vi "Asynchronous Logging Loop.vi"(10 "Input Data":T7 {"File Logging Specs"."File Node Ref" format="%.0x"}) -> ()   [LabVIEW 2019, in "Embedded Data Logger Engine.lvlib"]
uses:
  Embedded Data Logger Engine.lvlib
  File Logging Specification.ctl
  Group Logging Specification.ctl
  Group Buffer Data.ctl
  Property Specification.ctl
  <vilib>/NI VeriStand/Custom Device API/Custom Device Item Ref.ctl
  Shared/Segment Files By.ctl
  Asynchronous Logging Loop State.ctl
  Add to Flushed Data Size.vi
  <vilib>/NI VeriStand/Custom Device API/Custom Device API.lvlib
  Shared/Embedded Data Logger Shared.lvlib
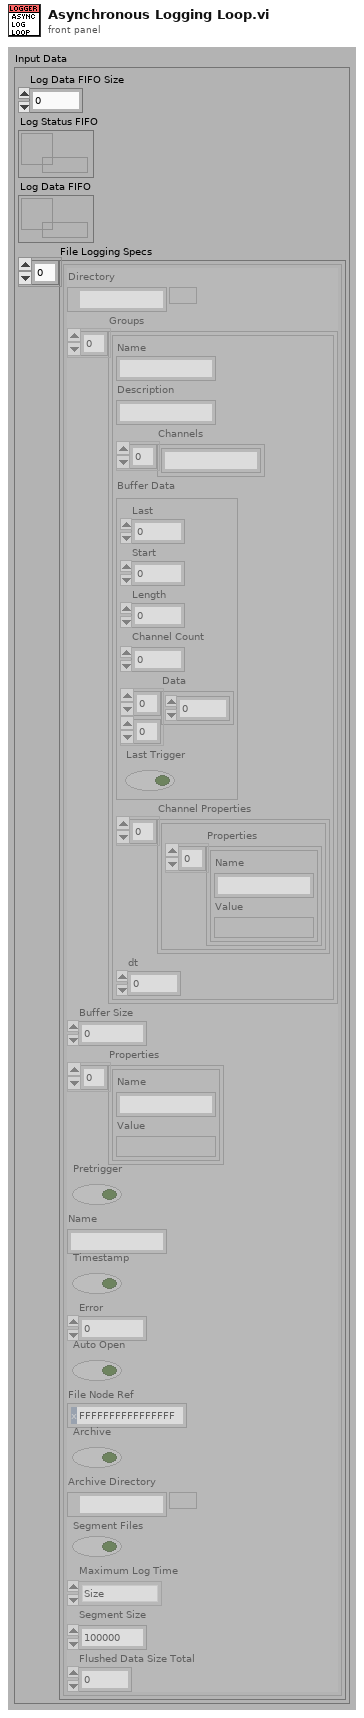
[diagram p1: front panel]
types:
  T1 = typedef "Embedded Data Logger Engine.lvlib/File Logging Specification.ctl" = cluster{"Directory":path, "Groups":T2[], "Buffer Size":i32, "Properties":T4[], "Pretrigger":bool, "Name":string, "Timestamp":bool, "Error":i32, "Auto Open":bool, "File Node Ref":T5, "Archive":bool, "Archive Directory":path, "Segment Files":bool, "Segment Files By":T6, "Segment Size":u32, "Flushed Data Size Total":u32}
  T2 = typedef "Embedded Data Logger Engine.lvlib/Group Logging Specification.ctl" = cluster{"Name":string, "Description":string, "Channels":string[], "Buffer Data":T3, "Channel Properties":cluster{"Properties":T4[]}[], "dt":dbl}
  T3 = typedef "Embedded Data Logger Engine.lvlib/Group Buffer Data.ctl" = cluster{"Last":i32, "Start":i32, "Length":i32, "Channel Count":i32, "Data":dbl[][], "Last Trigger":bool}
  T4 = typedef "Embedded Data Logger Engine.lvlib/Property Specification.ctl" = cluster{"Name":string, "Value":variant}
  T5 = typedef "Custom Device API.lvlib/Custom Device Item Ref.ctl" = u64
  T6 = typedef "Embedded Data Logger Shared.lvlib/Segment Files By.ctl" = enum16{"Time", "Size"}
  T7 = cluster{"Log Data FIFO Size":i32, "Log Status FIFO":refnum<k33>, "Log Data FIFO":refnum<k33>, "File Logging Specs":T1[]}
  T8 = typedef "Embedded Data Logger Engine.lvlib/Asynchronous Logging Loop State.ctl" = enum16{"Initialize", "Check Cmd", "Log Data", "Open File", "Close File", "Shut Down", "Open File then Log Data"}
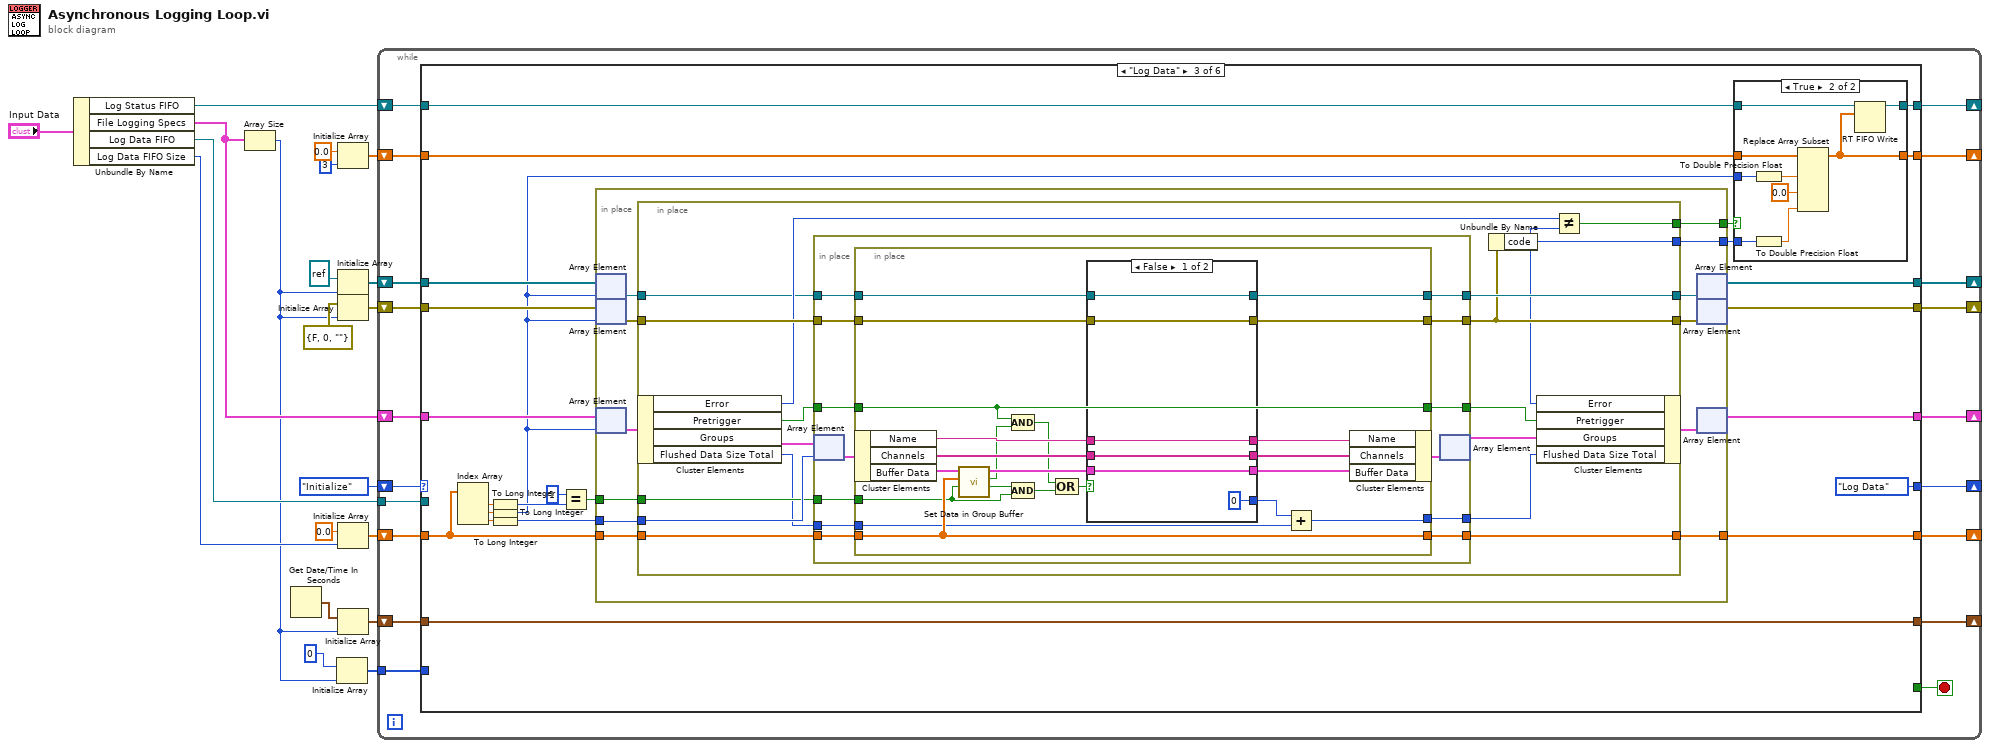
[diagram p0: block diagram]
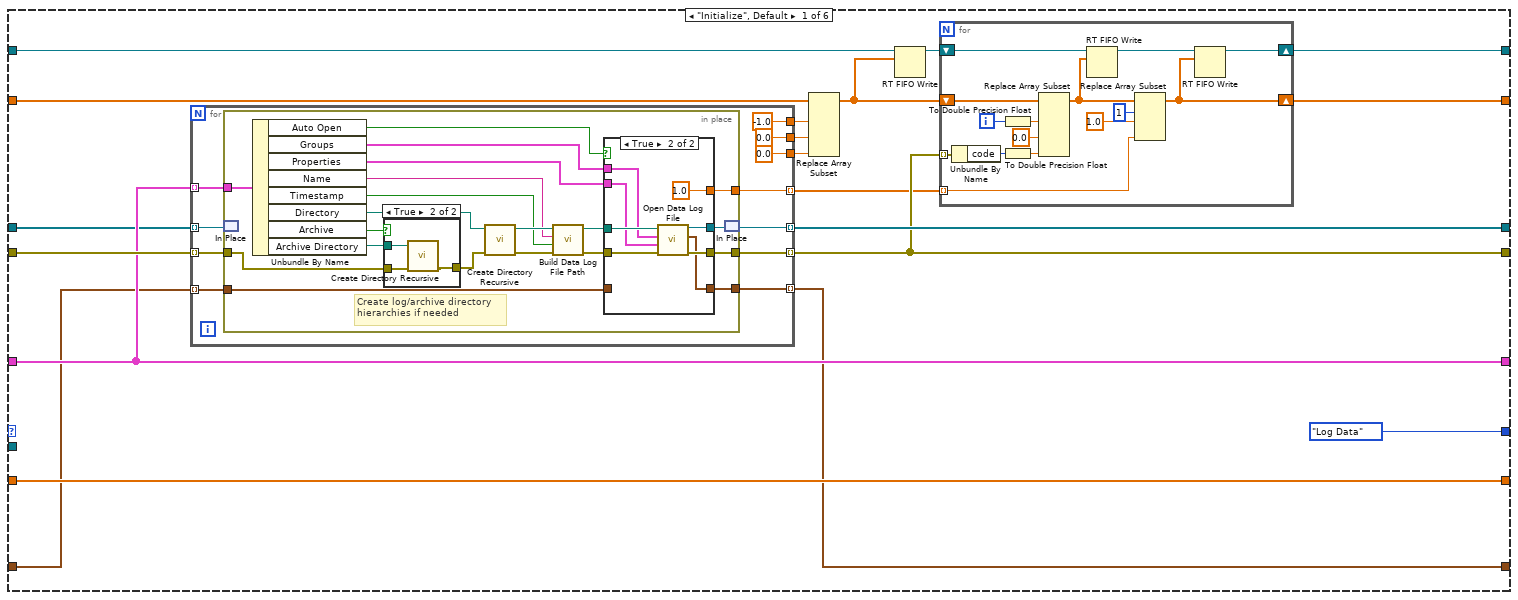
[diagram p2: hidden frame]
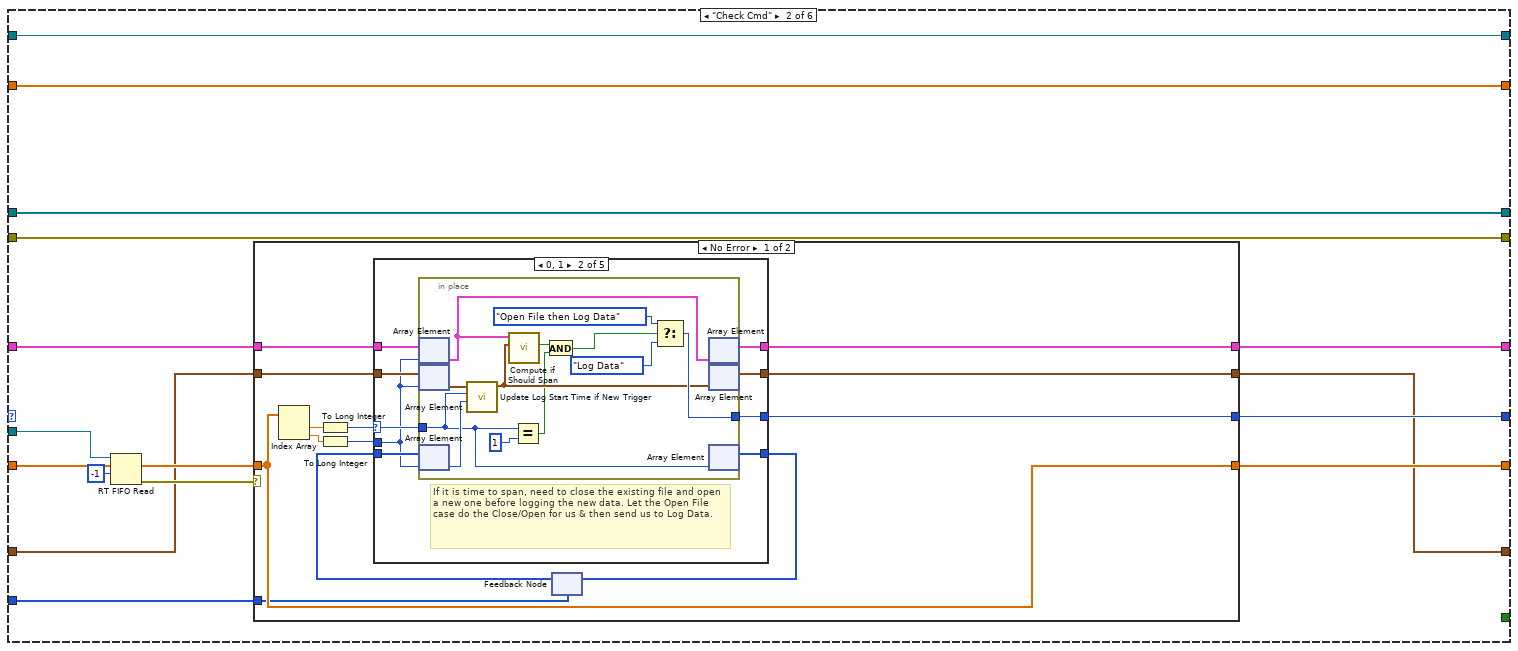
[diagram p5: hidden frame]
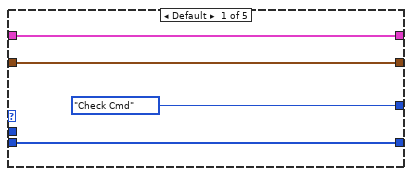
[diagram p6: hidden frame]
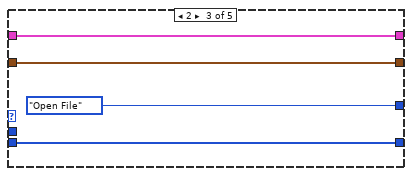
[diagram p7: hidden frame]
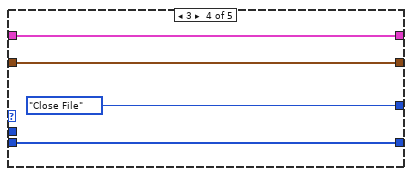
[diagram p8: hidden frame]
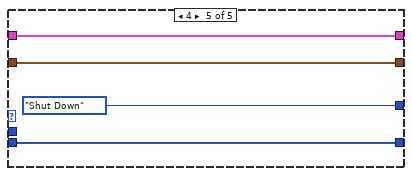
[diagram p9: hidden frame]
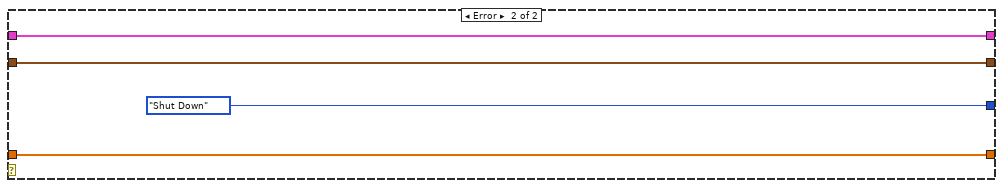
[diagram p10: hidden frame]
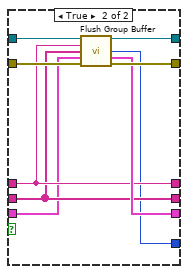
[diagram p11: hidden frame]
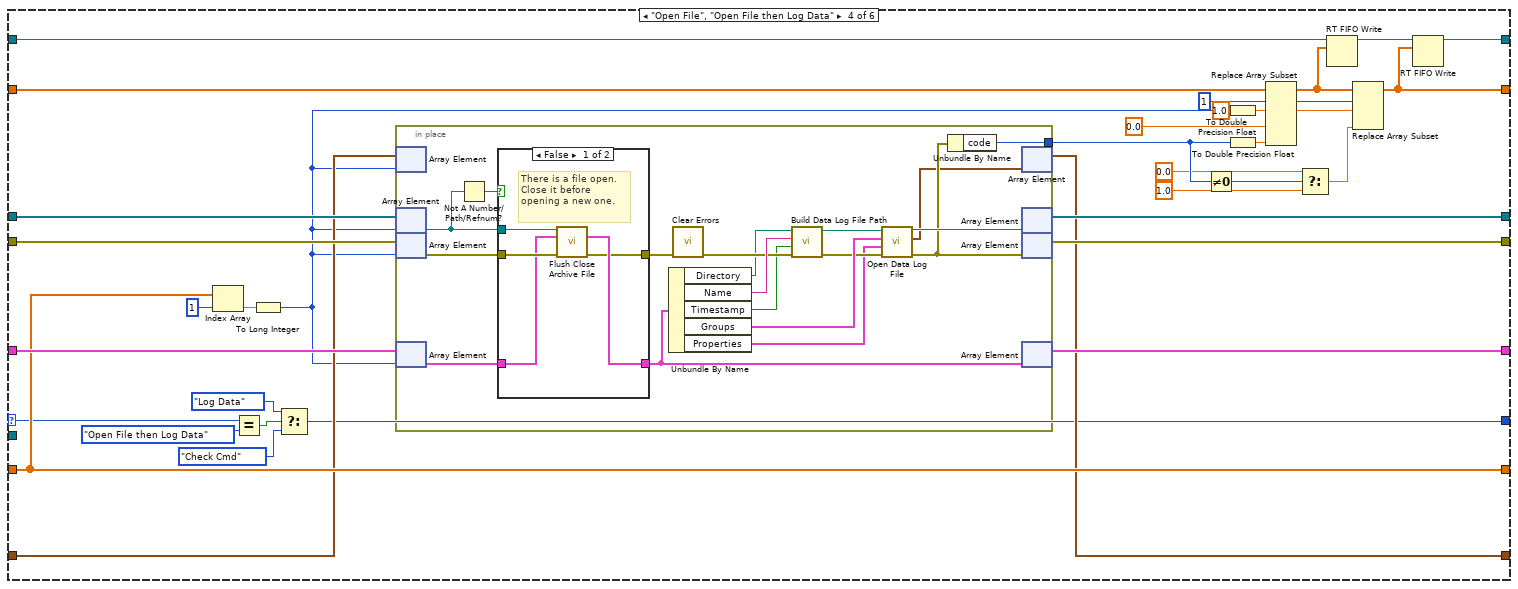
[diagram p13: hidden frame]
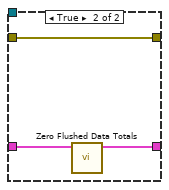
[diagram p14: hidden frame]
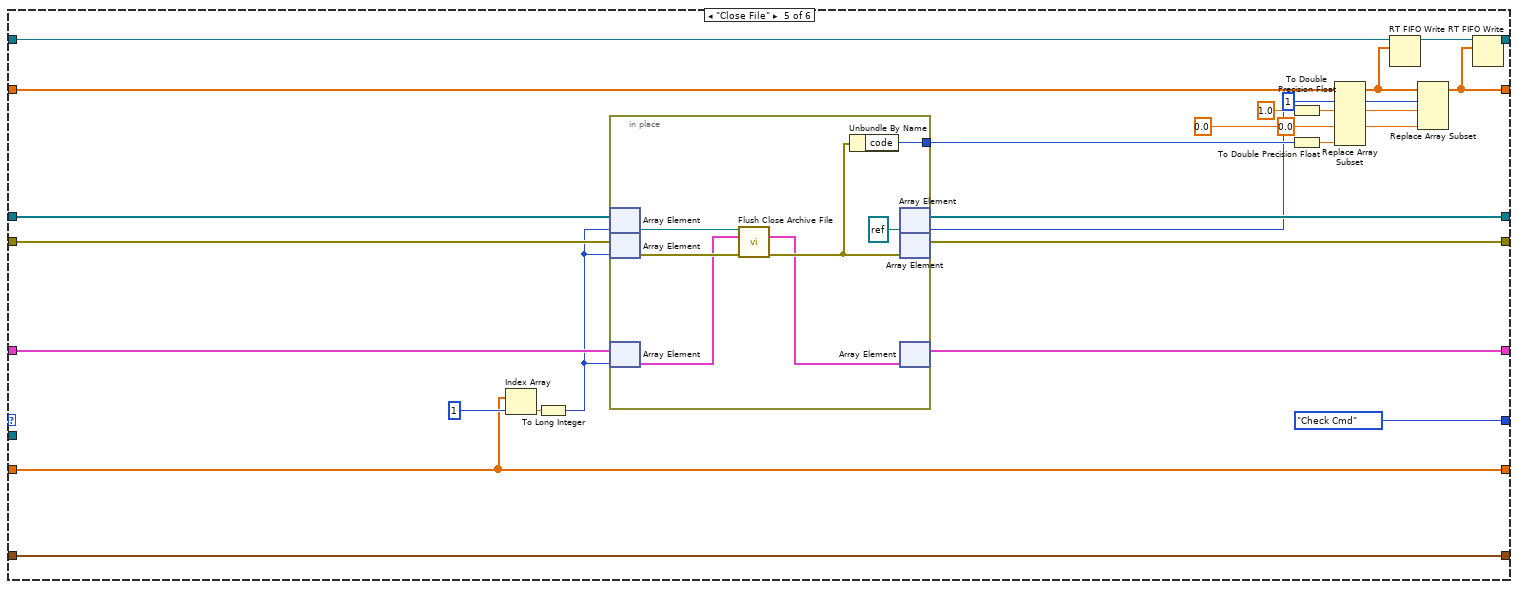
[diagram p15: hidden frame]
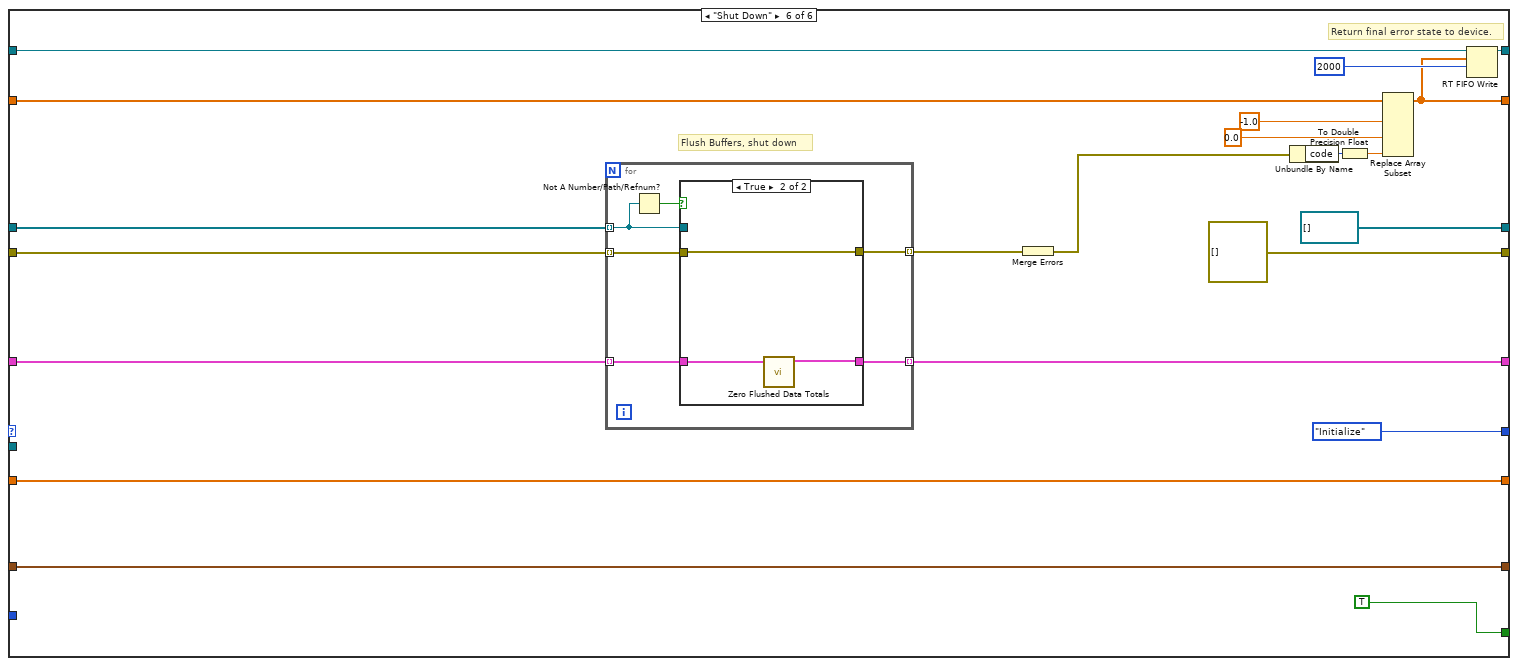
[diagram p16: hidden frame]
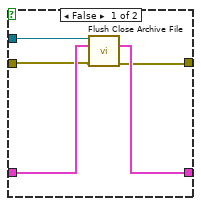
[diagram p17: hidden frame]
diagram:
  n1 = Unbundle By Name("Input Data") -> ("Log Status FIFO"=w14:refnum<k33>, "File Logging Specs"=w11:T1[], "Log Data FIFO"=w16:refnum<k33>, "Log Data FIFO Size"=w17:i32)
  n2 = Array Size(array=w11) -> (size(s)=w4:i32)
  n3 = Get Date/Time In Seconds() -> (seconds since 1Jan1904=w1:timestamp)
  n4 = Initialize Array(0 ("y"), w4) -> (w2:i32[])
  n5 = Initialize Array(0.0 ("element"), 3 ("dimension size")) -> (w6:dbl[])
  n6 = Initialize Array(refnum<k34> refnum ("TDMS File Ref out"), w4) -> (w9:refnum<k34>[])
  n7 = Initialize Array(errorcluster {"status"=FALSE, "code"=0, "source"=""} ("error in (no error)"), w4) -> (w12:errorcluster[])
  n8 = Initialize Array(0.0 ("element"), w17) -> (w19:dbl[])
  n9 = Initialize Array(w1, w4) -> (w5:timestamp[])
  n10 = while {
    tunnel: w16 -> [w39]
    shift-right: [w35] -> _
    shift-left: w19 -> [w38]
    shift-right: [w29] -> _
    shift-left: w9 -> [w28]
    shift-right: [w32] -> _
    shift-left: w11 -> [w33]
    shift-right: [w27] -> _
    shift-left: w14 -> [w26]
    shift-right: [w31] -> _
    shift-left: w12 -> [w30]
    shift-right: [w34] -> _
    shift-left: Asynchronous_Logging_Loop_State."Initialize" ("State") -> [w37]
    shift-right: [w24] -> _
    shift-left: w6 -> [w25]
    shift-right: [w22] -> _
    shift-left: w5 -> [w23]
    tunnel: w2 -> [w21]
    stop <- w36 stop-if-true
    n11 = case shown="\"Log Data\"" w37 {
      selector: w37 -> [_ _ _ w309 _ _]
      tunnel: w39 -> [_ w134 _ _ _ _]
      tunnel: w38 -> [w57 w120 w207 w328 w381 w413]
      tunnel: [_ _ _ _ _ TRUE] -> w36
      tunnel: [w57 w126 w196 w328 w381 w413] -> w35
      tunnel: [Asynchronous_Logging_Loop_State."Log Data" ("State") w125 Asynchronous_Logging_Loop_State."Log Data" ("State") w305 Asynchronous_Logging_Loop_State."Check Cmd" ("State") Asynchronous_Logging_Loop_State."Initialize" ("State")] -> w34
      tunnel: w33 -> [w54 w121 w202 w330 w367 w398]
      tunnel: [w54 w122 w197 w329 w364 w397] -> w32
      tunnel: [w51 w130 w198 w331 w383 errorcluster[] []] -> w31
      tunnel: w30 -> [w58 w130 w208 w332 w384 w414]
      tunnel: [w55 w129 w200 w333 w385 refnum<k34>[] []] -> w29
      tunnel: w28 -> [w50 w129 w209 w334 w386 w415]
      tunnel: [w45 w128 w199 w322 w372 w406] -> w27
      tunnel: w26 -> [w53 w128 w212 w324 w379 w399]
      tunnel: w25 -> [w49 w127 w191 w327 w378 w402]
      tunnel: [w44 w127 w192 w320 w368 w403] -> w24
      tunnel: w23 -> [w41 w123 w189 w311 w363 w396]
      tunnel: [w40 w124 w189 w310 w363 w396] -> w22
      tunnel: w21 -> [_ w119 _ _ _ _]
      frame "Initialize", Default {
        n12 = for {
          tunnel: w54 -> [w84] mode=indexing
          tunnel: [w81] -> w55 mode=indexing
          tunnel: [w82] -> w51 mode=indexing
          tunnel: w58 -> [w83] mode=indexing
          tunnel: w50 -> [w80] mode=indexing
          tunnel: [-1.0 ("new element/subarray")] -> w48
          tunnel: [0.0 ("new element/subarray")] -> w47
          tunnel: [w77] -> w43 mode=indexing
          tunnel: [0.0 ("new element/subarray")] -> w42
          tunnel: w41 -> [w74] mode=indexing
          tunnel: [w75] -> w40 mode=indexing
          n13 = in-place {
            in-place-border: w84 -> [w104]
            in-place-border: w83 -> [w90]
            in-place-border: [w96] -> w82
            in-place-border: [w93] -> w77
            in-place-border: [w86] -> w75
            in-place-border: w74 -> [w85]
            # "Create log/archive directory hierarchies if needed"
            n14 = in-place-match #1(w80) -> ()  [unwired: 1 out]
            n15 = Unbundle By Name(w104) -> ("Auto Open"=w94:bool, "Groups"=w97:T2[], "Properties"=w98:T4[], "Name"=w101:string, "Timestamp"=w100:bool, "Directory"=w88:path, "Archive"=w92:bool, "Archive Directory"=w89:path)
            n16 = case shown="True" w92 {
              tunnel: [w105 w108] -> w91
              tunnel: w90 -> [w105 w107]
              tunnel: w89 -> [_ w106]
              frame False {
              }
              frame True {
                n17 = call <vilib>:"Create Directory Recursive.vi"("error in (no error)"=w107, "directory"=w106) -> ("error out"=w108:errorcluster)  [unwired: 1 in, 4 out]
              }
            }
            n18 = call <vilib>:"Create Directory Recursive.vi"("error in (no error)"=w91, "directory"=w88) -> ("error out"=w103:errorcluster, "directory copy"=w102:path)  [unwired: 1 in, 3 out]
            n19 = call "Build Data Log File Path.vi"("error in (no error)"=w103, "Timestamp"=w100, "Name"=w101, "Log File Directory"=w102) -> ("error out"=w99:errorcluster, "appended path"=w87:path)  [unwired: 6 in]
            n20 = case shown="True" w94 {
              tunnel: w99 -> [w110 w118]
              tunnel: w87 -> [_ w117]
              tunnel: w98 -> [_ w116]
              tunnel: w97 -> [_ w115]
              tunnel: [w110 w114] -> w96
              tunnel: [_ w113] -> w95
              tunnel: [_ 1.0 ("new element/subarray")] -> w93
              tunnel: [w109 w111] -> w86
              tunnel: w85 -> [w109 _]
              frame False {
              }
              frame True {
                n21 = call "Open Data Log File.vi"("error in"=w118, "File Properties"=w116, "Channel Groups"=w115, "Data Log File Path"=w117) -> ("error out"=w114:errorcluster, "File Start Time"=w111:timestamp, "tdms file out"=w113:refnum<k34>)  [unwired: 5 in]
              }
            }
            n22 = in-place-match #1(w95) -> (w81:refnum<k34>)
          }
        }
        n23 = Replace Array Subset(array=w49, new element #1=w48, new element #2=w47, new element #3=w42) -> (w46:dbl[])  [unwired: 3 in]
        n24 = RT FIFO Write(0:w53, 1:w46) -> (8:w52:refnum<k33>)  [unwired: 2 in, 4 out]
        n25 = for {
          shift-right: [w63] -> w45
          shift-left: w52 -> [w73]
          tunnel: w51 -> [w71] mode=indexing
          shift-right: [w59] -> w44
          shift-left: w46 -> [w69]
          tunnel: w43 -> [w60] mode=indexing
          i -> [w72]
          n26 = Unbundle By Name(w71) -> ("code"=w70:i32)
          n27 = To Double Precision Float(number=w72) -> (double precision float=w66:dbl)
          n28 = To Double Precision Float(number=w70) -> (double precision float=w68:dbl)
          n29 = Replace Array Subset(array=w69, new element #1=w66, new element #2=0.0 ("new element/subarray"), new element #3=w68) -> (w67:dbl[])  [unwired: 3 in]
          n30 = RT FIFO Write(0:w73, 1:w67) -> (8:w64:refnum<k33>)  [unwired: 2 in, 4 out]
          n31 = Replace Array Subset(array=w67, new element #1=1.0 ("new element/subarray"), index #1=1 ("index"), new element #2=w60) -> (w59:dbl[])  [unwired: 1 in]
          n32 = RT FIFO Write(0:w64, 1:w59) -> (8:w63:refnum<k33>)  [unwired: 2 in, 4 out]
        }
      }
      frame "Check Cmd" {
        n33 = RT FIFO Read(0:w134, 1:w120, 2:-1 ("timeout in ms (0)")) -> (9:w131:dbl[], 11:w132:errorcluster)  [unwired: 1 in, 3 out]
        n34 = case shown="No Error" w132 {
          tunnel: [w138 w187] -> w126
          tunnel: w131 -> [w138 w187]
          tunnel: [w145 Asynchronous_Logging_Loop_State."Shut Down" ("State")] -> w125
          tunnel: w121 -> [w142 w186]
          tunnel: w123 -> [w141 w185]
          tunnel: [w140 w185] -> w124
          tunnel: [w139 w186] -> w122
          tunnel: w119 -> [w137 _]
          frame No Error {
            n35 = Index Array(array=w138) -> (element #1=w147:dbl, element #2=w144:dbl)  [unwired: 2 in]
            n36 = To Long Integer(number=w147) -> (32bit integer=w146:i32)
            n37 = To Long Integer(number=w144) -> (32bit integer=w143:i32)
            n38 = feedback #2(w137) -> (w136:i32[])
            n39 = case shown="0, 1" w146 {
              selector: w146 -> [_ w155 _ _ _]
              tunnel: [Asynchronous_Logging_Loop_State."Check Cmd" ("State") w158 Asynchronous_Logging_Loop_State."Open File" ("State") Asynchronous_Logging_Loop_State."Close File" ("State") Asynchronous_Logging_Loop_State."Shut Down" ("State")] -> w145
              tunnel: w143 -> [_ w153 _ _ _]
              tunnel: w142 -> [w149 w160 w175 w178 w182]
              tunnel: w141 -> [w150 w159 w174 w179 w183]
              tunnel: [w150 w157 w174 w179 w183] -> w140
              tunnel: [w149 w156 w175 w178 w182] -> w139
              tunnel: w136 -> [w148 w154 w173 w177 w181]
              tunnel: [w148 w152 w173 w177 w181] -> w135
              frame Default {
              }
              frame 0, 1 {
                # "If it is time to span, need to close the existing file and open a new one before logging the new data. Let the Open File case do the Close/Open for us & then send us to Log Data."
                n40 = in-place {
                  in-place-border: [w170] -> w158
                  in-place-border: w155 -> [w161]
                  n41 = in-place-array #3(w160, w153) -> (w169:T1)
                  n42 = in-place-array #4(w159, w153) -> (w166:timestamp)
                  n43 = in-place-array #5(w154, w153) -> (w162:i32)
                  n44 = call "Update Log Start Time if New Trigger.vi"("Previous Trigger Value"=w162, "Current Trigger Value"=w161, "Previous Log Trigger Time"=w166) -> ("Current Log Trigger Time"=w165:timestamp)  [unwired: 8 in]
                  n45 = call "Compute if Should Span.vi"("Log Start Time"=w165, "File Log Specification"=w169) -> ("Span File"=w168:bool)  [unwired: 9 in]
                  n46 = Equal?(x=w161, y=1) -> (x = y?=w163:bool)
                  n47 = And(x=w168, y=w163) -> (x .and. y?=w167:bool)
                  n48 = Select(t=Asynchronous_Logging_Loop_State."Open File then Log Data" ("State"), s=w167, f=Asynchronous_Logging_Loop_State."Log Data" ("State")) -> (s? t:f=w170:T8)
                  n49 = in-place-array #3(w169) -> (w156:T1[])  [unwired: 1 out]
                  n50 = in-place-array #4(w165) -> (w157:timestamp[])  [unwired: 1 out]
                  n51 = in-place-array #5(w161) -> (w152:i32[])  [unwired: 1 out]
                }
              }
              frame 2 {
              }
              frame 3 {
              }
              frame 4 {
              }
            }
            n52 = feedback-in #2(w135) -> ()
          }
          frame Error {
          }
        }
      }
      frame "Log Data" {
        n53 = Index Array(array=w207) -> (element #1=w206:dbl, element #2=w205:dbl, element #3=w204:dbl)  [unwired: 3 in]
        n54 = To Long Integer(number=w206) -> (32bit integer=w203:i32)
        n55 = To Long Integer(number=w205) -> (32bit integer=w190:i32)
        n56 = To Long Integer(number=w204) -> (32bit integer=w201:i32)
        n57 = Equal?(x=1, y=w203) -> (x = y?=w210:bool)
        n58 = in-place {
          in-place-border: w207 -> [w224]
          in-place-border: w201 -> [w223]
          in-place-border: w210 -> [w221]
          in-place-border: [w218] -> w196
          in-place-border: [w215] -> w194
          in-place-border: [w214] -> w193
          n59 = in-place-array #6(w209, w190) -> (w220:refnum<k34>)
          n60 = in-place-array #7(w208, w190) -> (w217:errorcluster)
          n61 = in-place-array #8(w202, w190) -> (w222:T1)
          n62 = in-place {
            in-place-border: w224 -> [w239]
            in-place-border: w223 -> [w238]
            in-place-border: w221 -> [w235]
            in-place-border: w217 -> [w241]
            in-place-border: [w229] -> w216
            in-place-border: w220 -> [w234]
            in-place-border: [w233] -> w219
            in-place-border: [w232] -> w218
            in-place-border: [w228] -> w215
            in-place-border: [w227] -> w214
            n63 = in-place-cluster #9(w222) -> ("Error"=w240:i32, "Pretrigger"=w231:bool, "Groups"=w237:T2[], "Flushed Data Size Total"=w226:u32)
            n64 = in-place {
              in-place-border: w239 -> [w254]
              in-place-border: w235 -> [w251]
              in-place-border: w241 -> [w250]
              in-place-border: [w249] -> w229
              in-place-border: w234 -> [w248]
              in-place-border: [w247] -> w233
              in-place-border: [w246] -> w232
              in-place-border: w231 -> [w245]
              in-place-border: [w244] -> w230
              in-place-border: w226 -> [w243]
              in-place-border: [w242] -> w225
              n65 = in-place-array #10(w237, w238) -> (w253:T2)
              n66 = in-place {
                in-place-border: w254 -> [w264]
                in-place-border: w251 -> [w263]
                in-place-border: w250 -> [w276]
                in-place-border: [w270] -> w249
                in-place-border: w248 -> [w265]
                in-place-border: [w266] -> w247
                in-place-border: [w264] -> w246
                in-place-border: w245 -> [w259]
                in-place-border: [w259] -> w244
                in-place-border: w243 -> [w257]
                in-place-border: [w256] -> w242
                n67 = in-place-cluster #11(w253) -> ("Name"=w271:string, "Channels"=w269:string[], "Buffer Data"=w275:T3)
                n68 = call "Set Data in Group Buffer.vi"("New Trigger"=w263, "Data in"=w264, "Group Buffer Data in"=w275) -> ("Buffer Full"=w274:bool, "Flush Pretrigger Data"=w262:bool, "Group Buffer Data out"=w272:T3)  [unwired: 6 out]
                n69 = Compound Arithmetic op=AND(w259, w262) -> (w260:bool)
                n70 = Compound Arithmetic op=AND(w274, w263) -> (w273:bool)
                n71 = Compound Arithmetic op=OR(w260, w273) -> (w261:bool)
                n72 = case shown="False" w261 {
                  tunnel: w272 -> [w282 w284]
                  tunnel: w271 -> [w280 w286]
                  tunnel: [w282 w289] -> w258
                  tunnel: w276 -> [w281 w291]
                  tunnel: [w281 w290] -> w270
                  tunnel: w269 -> [w279 w285]
                  tunnel: [w280 w286] -> w268
                  tunnel: [w279 w285] -> w267
                  tunnel: [w278 w287] -> w266
                  tunnel: w265 -> [w278 w288]
                  tunnel: [u32 0 ("Flushed Data Size") w283] -> w255
                  frame False {
                  }
                  frame True {
                    n73 = call "Flush Group Buffer.vi"("TDMS File Ref in"=w288, "Group Name"=w286, "Channels"=w285, "Group Buffer Data in"=w284, "error in (no error)"=w291) -> ("TDMS File Ref out"=w287:refnum<k34>, "Flushed Data Size"=w283:u32, "Group Buffer Data out"=w289:T3, "error out"=w290:errorcluster)  [unwired: 1 in, 6 out]
                  }
                }
                n74 = Add(x=w255, y=w257) -> (x+y=w256:u32)
                n75 = in-place-cluster #11("Name"=w268, "Channels"=w267, "Buffer Data"=w258) -> (w252:T2)
              }
              n76 = in-place-array #10(w252) -> (w236:T2[])  [unwired: 1 out]
            }
            n77 = Unbundle By Name(w229) -> ("code"=w228:i32)
            n78 = in-place-cluster #9("Error"=w228, "Pretrigger"=w230, "Groups"=w236, "Flushed Data Size Total"=w225) -> (w213:T1)
            n79 = Not Equal?(x=w240, y=w228) -> (x != y?=w227:bool)
          }
          n80 = in-place-array #6(w219) -> (w200:refnum<k34>[])  [unwired: 1 out]
          n81 = in-place-array #7(w216) -> (w198:errorcluster[])  [unwired: 1 out]
          n82 = in-place-array #8(w213) -> (w197:T1[])  [unwired: 1 out]
        }
        n83 = case shown="True" w193 {
          tunnel: w212 -> [w293 w302]
          tunnel: w190 -> [_ w301]
          tunnel: [w293 w300] -> w199
          tunnel: w194 -> [_ w299]
          tunnel: [w292 w297] -> w192
          tunnel: w191 -> [w292 w298]
          frame False {
          }
          frame True {
            n84 = To Double Precision Float(number=w301) -> (double precision float=w295:dbl)
            n85 = To Double Precision Float(number=w299) -> (double precision float=w296:dbl)
            n86 = Replace Array Subset(array=w298, new element #1=w295, new element #2=0.0 ("new element/subarray"), new element #3=w296) -> (w297:dbl[])  [unwired: 3 in]
            n87 = RT FIFO Write(0:w302, 1:w297) -> (8:w300:refnum<k33>)  [unwired: 2 in, 4 out]
          }
        }
      }
      frame "Open File", "Open File then Log Data" {
        n88 = Index Array(array=w328, index=1) -> (element=w336:dbl)
        n89 = Equal?(x=w309, y=Asynchronous_Logging_Loop_State."Open File then Log Data" ("State")) -> (x = y?=w304:bool)
        n90 = To Long Integer(number=w336) -> (32bit integer=w303:i32)
        n91 = Select(t=Asynchronous_Logging_Loop_State."Log Data" ("State"), s=w304, f=Asynchronous_Logging_Loop_State."Check Cmd" ("State")) -> (s? t:f=w305:T8)
        n92 = in-place {
          in-place-border: [w348] -> w316
          n93 = in-place-array #12(w311, w303) -> ()  [unwired: 1 out]
          n94 = in-place-array #13(w334, w303) -> (w343:refnum<k34>)
          n95 = in-place-array #14(w332, w303) -> (w350:errorcluster)
          n96 = in-place-array #15(w330, w303) -> (w341:T1)
          n97 = Not A Number/Path/Refnum?(number/path/refnum=w343) -> (NaN/Path/Refnum?=w342:bool)
          n98 = case shown="False" w342 {
            tunnel: w350 -> [w358 w362]
            tunnel: [w355 w362] -> w349
            tunnel: w343 -> [w359 _]
            tunnel: [w356 w360] -> w337
            tunnel: w341 -> [w357 w361]
            frame False {
              # "There is a file open. Close it before opening a new one."
              n99 = call "Flush Close Archive File.vi"("TDMS File Refnum In"=w359, "File Log Spec In"=w357, "error in"=w358) -> ("File Log Spec Out"=w356:T1, "error out"=w355:errorcluster)  [unwired: 11 in]
            }
            frame True {
              n100 = call "Zero Flushed Data Totals.vi"("File Log Spec in"=w361) -> ("File Log Spec out"=w360:T1)  [unwired: 10 in]
            }
          }
          n101 = Unbundle By Name(w337) -> ("Directory"=w346:path, "Name"=w354:string, "Timestamp"=w345:bool, "Groups"=w353:T2[], "Properties"=w344:T4[])
          n102 = call <vilib>:"Clear Errors.vi"("error in (no error)"=w349) -> ("error out"=w347:errorcluster)  [unwired: 5 in, 1 out]
          n103 = call "Build Data Log File Path.vi"("error in (no error)"=w347, "Timestamp"=w345, "Name"=w354, "Log File Directory"=w346) -> ("error out"=w352:errorcluster, "appended path"=w340:path)  [unwired: 6 in]
          n104 = call "Open Data Log File.vi"("error in"=w352, "File Properties"=w344, "Channel Groups"=w353, "Data Log File Path"=w340) -> ("error out"=w339:errorcluster, "File Start Time"=w338:timestamp, "tdms file out"=w351:refnum<k34>)  [unwired: 5 in]
          n105 = Unbundle By Name(w339) -> ("code"=w348:i32)
          n106 = in-place-array #12(w338) -> (w310:timestamp[])  [unwired: 1 out]
          n107 = in-place-array #13(w351) -> (w333:refnum<k34>[])  [unwired: 1 out]
          n108 = in-place-array #14(w339) -> (w331:errorcluster[])  [unwired: 1 out]
          n109 = in-place-array #15(w337) -> (w329:T1[])  [unwired: 1 out]
        }
        n110 = Not Equal To 0?(x=w316) -> (x != 0?=w315:bool)
        n111 = To Double Precision Float(number=w303) -> (double precision float=w319:dbl)
        n112 = To Double Precision Float(number=w316) -> (double precision float=w326:dbl)
        n113 = Replace Array Subset(array=w327, new element #1=w319, new element #2=0.0 ("new element/subarray"), new element #3=w326) -> (w321:dbl[])  [unwired: 3 in]
        n114 = Select(t=0.0, s=w315, f=1.0 ("new element/subarray")) -> (s? t:f=w312:dbl)
        n115 = RT FIFO Write(0:w324, 1:w321) -> (8:w323:refnum<k33>)  [unwired: 2 in, 4 out]
        n116 = Replace Array Subset(array=w321, new element #1=1.0 ("new element/subarray"), index #1=1 ("index"), new element #2=w312) -> (w320:dbl[])  [unwired: 1 in]
        n117 = RT FIFO Write(0:w323, 1:w320) -> (8:w322:refnum<k33>)  [unwired: 2 in, 4 out]
      }
      frame "Close File" {
        n118 = Index Array(array=w381, index=1) -> (element=w388:dbl)
        n119 = To Long Integer(number=w388) -> (32bit integer=w366:i32)
        n120 = in-place {
          in-place-border: [w395] -> w380
          n121 = in-place-array #16(w386, w366) -> (w392:refnum<k34>)
          n122 = in-place-array #17(w384, w366) -> (w393:errorcluster)
          n123 = in-place-array #18(w367, w366) -> (w391:T1)
          n124 = call "Flush Close Archive File.vi"("TDMS File Refnum In"=w392, "File Log Spec In"=w391, "error in"=w393) -> ("File Log Spec Out"=w389:T1, "error out"=w390:errorcluster)  [unwired: 11 in]
          n125 = Unbundle By Name(w390) -> ("code"=w395:i32)
          n126 = in-place-array #16(refnum<k34> refnum ("element")) -> (w385:refnum<k34>[], w365:i32)
          n127 = in-place-array #17(w390) -> (w383:errorcluster[])  [unwired: 1 out]
          n128 = in-place-array #18(w389) -> (w364:T1[])  [unwired: 1 out]
        }
        n129 = To Double Precision Float(number=w365) -> (double precision float=w375:dbl)
        n130 = To Double Precision Float(number=w380) -> (double precision float=w376:dbl)
        n131 = Replace Array Subset(array=w378, new element #1=w375, new element #2=0.0 ("new element/subarray"), new element #3=w376) -> (w377:dbl[])  [unwired: 3 in]
        n132 = RT FIFO Write(0:w379, 1:w377) -> (8:w373:refnum<k33>)  [unwired: 2 in, 4 out]
        n133 = Replace Array Subset(array=w377, new element #1=1.0 ("new element/subarray"), index #1=1 ("index"), new element #2=0.0 ("new element/subarray")) -> (w368:dbl[])  [unwired: 1 in]
        n134 = RT FIFO Write(0:w373, 1:w368) -> (8:w372:refnum<k33>)  [unwired: 2 in, 4 out]
      }
      frame "Shut Down" {
        # "Return final error state to device."
        # "Flush Buffers, shut down"
        n135 = for {
          tunnel: w398 -> [w421] mode=indexing
          tunnel: w415 -> [w419] mode=indexing
          tunnel: w414 -> [w422] mode=indexing
          tunnel: [w420] -> w405 mode=indexing
          tunnel: [w417] -> w397 mode=indexing
          n136 = Not A Number/Path/Refnum?(number/path/refnum=w419) -> (NaN/Path/Refnum?=w418:bool)
          n137 = case shown="True" w418 {
            tunnel: w422 -> [w425 w430]
            tunnel: w421 -> [w426 w429]
            tunnel: [w423 w430] -> w420
            tunnel: w419 -> [w427 _]
            tunnel: [w424 w428] -> w417
            frame False {
              n138 = call "Flush Close Archive File.vi"("TDMS File Refnum In"=w427, "File Log Spec In"=w426, "error in"=w425) -> ("File Log Spec Out"=w424:T1, "error out"=w423:errorcluster)  [unwired: 11 in]
            }
            frame True {
              n139 = call "Zero Flushed Data Totals.vi"("File Log Spec in"=w429) -> ("File Log Spec out"=w428:T1)  [unwired: 10 in]
            }
          }
        }
        n140 = Merge Errors(w405) -> (w404:errorcluster)
        n141 = Unbundle By Name(w404) -> ("code"=w407:i32)
        n142 = To Double Precision Float(number=w407) -> (double precision float=w410:dbl)
        n143 = Replace Array Subset(array=w402, new element #1=-1.0 ("new element/subarray"), new element #2=0.0 ("new element/subarray"), new element #3=w410) -> (w403:dbl[])  [unwired: 3 in]
        n144 = RT FIFO Write(0:w399, 1:w403, 2:2000 ("timeout in ms (0)")) -> (8:w406:refnum<k33>)  [unwired: 2 in, 3 out]
      }
    }
  }
